vi "Single Tone Audio Measurements.vi"(6 "units settings":T1, 8 "error in":errorcluster, 10 "measurement settings":T4={"Band start"=20.0, "Band stop"=20000.0, "Amplitude"=1.0, "Frequency"=1000.0, "Full scale range"=3.16, "Channel name"="0L"}, 11 "waveform":waveform(dbl)) -> (0 "error out":errorcluster, 1 "spectrum":cluster{"x0":dbl, "dx":dbl, "magnitude":dbl[]}, 2 "time domain":waveform(dbl), 3 "results":T5)   [LabVIEW 2021]
uses:
  controls/single tone audio measurements.ctl
  controls/single tone audio measurement settings.ctl
  <vilib>/addons/_NISVFA/_Shared subVIs/Common/SVL Set dB Reference (variant).vi
  <vilib>/addons/_NISVFA/_Spectrum Processing/SVFA Get Spectrum Subset.vi
  <vilib>/addons/_NISVFA/_Spectrum Processing/SVFA Get Spectrum Subset (Complex) (1 Ch).vi
  <vilib>/addons/_NISVFA/_Shared subVIs/Common/svc_Window Parameters.vi
  <vilib>/addons/_NISVFA/_Shared subVIs/Common/svc_Extract Single Tone Information (complex).vi
  <vilib>/addons/_NISVFA/_Shared subVIs/Common/svc_Check Frequency Range in Spectrum.vi
  <vilib>/addons/_NISVFA/_Spectrum Processing/SVFA Spectrum Peak Search.vi
  <vilib>/addons/_NISVFA/_Spectrum Processing/SVFA Spectrum Peak Search (1 Ch).vi
  <vilib>/addons/_NISVFA/_Shared subVIs/Common/svc_Spectrum Units.vi
  <vilib>/addons/_NISVFA/_Shared subVIs/Common/svc_Log View for Spectrum (1Ch).vi
  <vilib>/addons/_NISVFA/_Spectrum Processing/SVFA Unit Conversion (1 Ch).vi
  <vilib>/addons/_NISVFA/_Shared subVIs/Common/svc_Complex Datatype Defaults.vi
  <vilib>/addons/_NISVFA/_Shared subVIs/Common/svc_Build Unit Label for Frequency Range.vi
  <vilib>/addons/_NISVFA/_Spectrum Processing/SVFA Get Tone Amplitude and Phase (1 Ch).vi
  <vilib>/addons/_NISVFA/_Spectrum Processing/subVIs/svfa_Compute Complex Spectrum for Export.vi
  <vilib>/addons/_NISVFA/_Shared subVIs/Common/svc_Check Frequency Range in Bandwidth.vi
  <vilib>/addons/_NISVFA/_Shared subVIs/Common/svc_Convert Start and Stop to Start Index and Length.vi
  <vilib>/addons/_NISVFA/_Spectrum Processing/subVIs/svfa_Spectrum Peak Search.vi
  <vilib>/addons/_NISVFA/_Shared subVIs/Common/svc_Format Value (DBL).vi
  <vilib>/addons/_NISVFA/_Shared subVIs/Common/svc_Get Weighting Enum and Labels.vi
  <vilib>/addons/_NISVFA/_Shared subVIs/Common/svc_Engineering Units to Unit Label.vi
  <vilib>/addons/_NISVFA/_Shared subVIs/Common/svc_Surround NonAlpha String with Parentheses.vi
  <vilib>/dlg_ctls.llb/Space Constant.vi
  <vilib>/addons/_NISVFA/_Shared subVIs/Common/svc_Unwrap Phase.vi
  <vilib>/addons/_NISVFA/_Shared subVIs/Common/svc_Convert Spectrum Array to dB.vi
  <vilib>/addons/_NISVFA/_Spectrum Processing/subVIs/svfa_Conversion Utility (spectrum info).vi
  <vilib>/addons/_NISVFA/_Spectrum Processing/subVIs/svfa_Window Frequency Response.vi
  <vilib>/addons/_NISVFA/_Spectrum Processing/subVIs/svfa_Window Frequency Response (double array).vi
  <vilib>/Analysis/baseanly.llb/Dot Product.vi
  <vilib>/Analysis/baseanly.llb/Complex Dot Product.vi
  <vilib>/addons/_NISVFA/_Spectrum Processing/subVIs/svfa_Peak Rough Search Indices.vi
  <vilib>/addons/_NISVFA/_Shared subVIs/Common/svc_Unit Label Lexical Class.vi
  <vilib>/addons/_NISVFA/_Spectrum Processing/subVIs/svfa_Peak to RMS to Peak2Peak.vi
  <vilib>/addons/_NISVFA/_Spectrum Processing/subVIs/svfa_Mag to Mag2.vi
  <vilib>/addons/_NISVFA/_Spectrum Processing/subVIs/svfa_Linear to dB.vi
  <vilib>/addons/_NISVFA/_Spectrum Processing/subVIs/svfa_dBrefA to dBrefB.vi
  <vilib>/addons/_NISVFA/_Spectrum Processing/subVIs/svfa_Spectrum to Spectral Density.vi
  <vilib>/addons/_NISVFA/_Spectrum Processing/subVIs/svfa_Rect Window Frequency Response.vi
  <vilib>/addons/_NISVFA/_Spectrum Processing/subVIs/svfa_Cosine Window Coefficients.vi
  <vilib>/addons/_NISVFA/_Shared subVIs/Common/svc_Caller VI Returned in Error Source.vi
  <vilib>/addons/Sound and Vibration/svt_Distortion/subVIs/sv_Check Data Valid (Audio) (1 Ch).vi
  <vilib>/addons/_NISVFA/_Shared subVIs/Common/svc_Convert Frequency to Frequency String.vi
  <vilib>/Analysis/4window.llb/window parameters.vi
  <vilib>/Analysis/4window.llb/Window Properties.vi
  <vilib>/Analysis/4window.llb/Window Properties by Name.vi
  <vilib>/addons/_NISVFA/_Spectrum Processing/subVIs/svfa_Spectrum Peak Tone Search and Estimation (complex).vi
  <vilib>/measure/masignal.llb/Tones and Noise Waveform.vi
  <vilib>/addons/_NISVFA/_Shared subVIs/Common/svc_FFT with Window.vi
  <vilib>/Analysis/1siggen.llb/Square Wave.vi
  <vilib>/addons/_NISVFA/_Spectrum Processing/subVIs/svfa_Three Finger Peak Search.vi
  <vilib>/addons/Sound and Vibration/svt_Distortion/subVIs/sv_Peak View Amplitude (1 Ch).vi
  <vilib>/addons/Sound and Vibration/svt_Single Tone Measurements/SVT Gain (Time) (1 Ch).vi
  <vilib>/addons/Sound and Vibration/svt_Distortion/SVT SNR without Harmonics (Frequency) (1 Ch).vi
  <vilib>/addons/_NISVFA/_Shared subVIs/Common/SVL Set dB Reference (1 Ch).vi
  <vilib>/addons/_NISVFA/_Spectrum Processing/SVFA Unit Conversion (Complex) (1 Ch).vi
  <vilib>/addons/Sound and Vibration/svt_Single Tone Measurements/SVT Spurious Free Dynamic Range (Frequency) (1 Ch).vi
  <vilib>/addons/Sound and Vibration/svt_Single Tone Measurements/SVT Dynamic Range (Frequency) (1 Ch).vi
  <vilib>/addons/Sound and Vibration/svt_Single Tone Measurements/SoundVib_SingleTone.lvlib
  <vilib>/addons/Sound and Vibration/svt_Distortion/SoundVib_Distortion.lvlib
  controls/audio controls.lvlib
  controls/units - ratio.ctl
  controls/units - snr.ctl
  controls/units settings.ctl
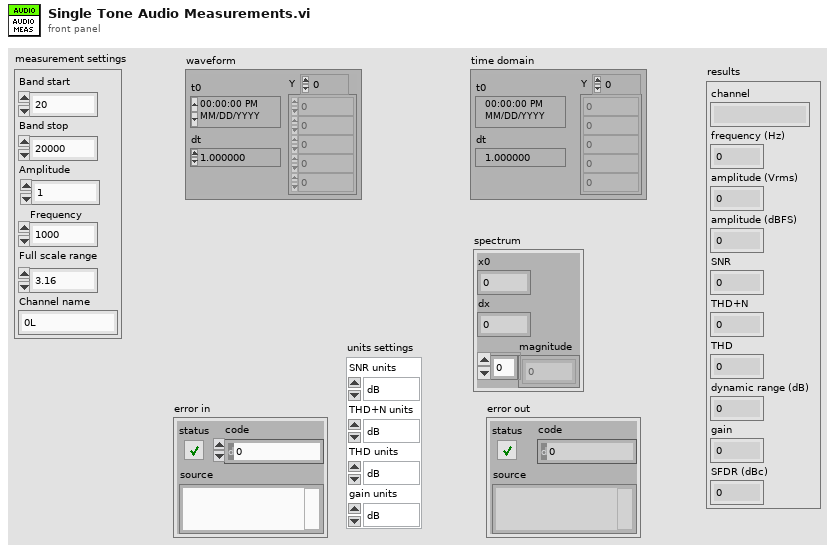
[diagram p1: front panel]
types:
  T1 = typedef "audio controls.lvlib/units settings.ctl" = cluster{"SNR units":T2, "THD+N units":T3, "THD units":T3, "gain units":T3}
  T2 = typedef "audio controls.lvlib/units - snr.ctl" = enum16{"dB", "x/y"}
  T3 = typedef "audio controls.lvlib/units - ratio.ctl" = enum16{"dB", "%", "x/y", "ppm"}
  T4 = typedef "audio controls.lvlib/single tone audio measurement settings.ctl" = cluster{"Band start":dbl, "Band stop":dbl, "Amplitude":dbl, "Frequency":dbl, "Full scale range":dbl, "Channel name":string}
  T5 = typedef "audio controls.lvlib/single tone audio measurements.ctl" = cluster{"channel":string, "frequency (Hz)":dbl, "amplitude (Vrms)":dbl, "amplitude (dBFS)":dbl, "SNR":dbl, "THD+N":dbl, "THD":dbl, "dynamic range (dB)":dbl, "gain":dbl, "SFDR (dBc)":dbl}
  T6 = enum16{"no change", "spectrum", "spectral density"}
  T7 = cluster{"linear/dB":enum16{"no change", "linear", "dB"}, "dB reference (0: no change)":dbl, "power/magnitude":enum16{"no change", "power", "magnitude"}, "view":enum16{"no change", "rms", "peak", "peak-peak"}}
  T8 = cluster{"start frequency":dbl, "stop frequency":dbl}
  T9 = cluster{"gain units":enum16{"dB", "linear ratio"}, "detected fundamental amplitude units":enum16{"EU rms", "EU peak", "EU peak-peak"}}
  T10 = cluster{"SNR units":enum16{"dB", "linear ratio", "%"}, "detected fundamental amplitude units":enum16{"EU rms", "EU peak", "EU peak-peak"}}
  T11 = typedef "svc_Spectrum Info.ctl" = cluster{"channel name":string, "description":string, "x-axis units":T12, "spectral info":cluster{"spectrum type":T13, "linear/dB":enum16{"linear", "dB"}, "window":u16, "window size":i32, "FFT size":i32}, "engineering units":T14, "custom label":string, "dB reference [EU]":dbl, "peak units":enum16{"rms", "peak", "peak-peak"}, "weighting filter":T15, "spectral density?":bool, "unit label":string, "spectrum skewed?":bool, "complimentary spectrum units":T16}
  T12 = typedef "svc_X-Axis Units.ctl" = u16
  T13 = typedef "svc_Spectrum Type.ctl" = enum16{"FFT Spectrum [complex]", "Amplitude [Magnitude]", "Power [Magnitude^2]", "Cross Spectrum [complex]", "Frequency Response [Complex]"}
  T14 = typedef "svc_Engineering Units Text Ring.ctl" = u16
  T15 = typedef "svc_Weighting Filter Text Ring.ctl" = u16
  T16 = typedef "svc_Complimentary Spectrum Units.ctl" = enum16{"none", "radians", "degrees", "cycles", "imaginary"}
  T17 = cluster{"complex spectrum response":cluster{"f0":dbl, "df":dbl, "complex spectrum":cdb[]}, "spectrum info":T11}
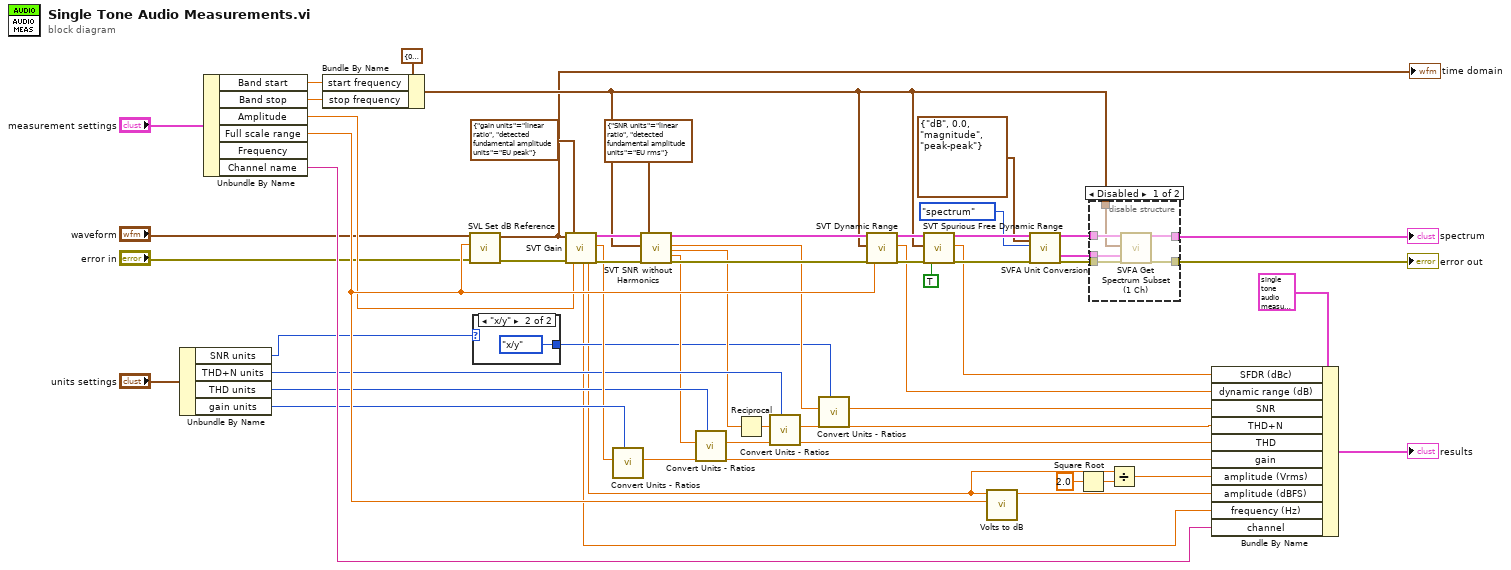
[diagram p0: block diagram]
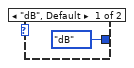
[diagram p2: hidden frame]
diagram:
  n1 = Unbundle By Name("units settings") -> ("SNR units"=w8:T2, "THD+N units"=w17:T3, "THD units"=w11:T3, "gain units"=w20:T3)
  n2 = Unbundle By Name("measurement settings") -> ("Band start"=w54:dbl, "Band stop"=w55:dbl, "Amplitude"=w26:dbl, "Full scale range"=w33:dbl, "Channel name"=w25:string)  [unwired: 1 out]
  n3 = Bundle By Name(cluster=T8 {"start frequency"=0.0, "stop frequency"=0.0} ("frequency range"), "start frequency"=w54, "stop frequency"=w55) -> (w38:T8)
  n4 = call-poly <vilib>:"SVL Set dB Reference.vi"("error in (no error)"="error in", "dB reference [EU]"=w33, "scaled signal in [EU]"="waveform") -> ("error out"=w27:errorcluster, "scaled signal out [EU]"=w23:waveform(dbl))  [unwired: 7 in]
  "time domain" <- w23
  n5 = case shown="\"x/y\"" w8 {
    tunnel: [units_-_ratio."dB" ("gain units") units_-_ratio."x/y" ("gain units")] -> w7
    frame "dB", Default {
    }
    frame "x/y" {
    }
  }
  n6 = call-poly <vilib>:"SVT Gain.vi"("scaled signal [EU]"=w23, "error in (no error)"=w27, "desired units"=T9 {"gain units"=enum."linear ratio", "detected fundamental amplitude units"=enum."EU peak"}, "amplitude [EU peak]"=w26) -> ("detected fundamental\nfrequency [Hz]"=w6:dbl, "detected fundamental\namplitude"=w1:dbl, "complex spectrum"=w44:T17, "gain"=w19:dbl, "error out"=w45:errorcluster)  [unwired: 10 in, 1 out]
  n7 = call "Convert Units - Ratios.vi"("gain units"=w20, "linear ratio"=w19) -> ("converted ratio"=w18:dbl)  [unwired: 9 in]
  n8 = call-poly <vilib>:"SVT SNR without Harmonics.vi"("complex spectrum"=w44, "frequency range"=w38, "error in (no error)"=w45, "desired units"=T10 {"SNR units"=enum."linear ratio", "detected fundamental amplitude units"=enum."EU rms"}) -> ("complex spectrum"=w47:T17, "SNR (without harmonics)"=w16:dbl, "SINAD"=w13:dbl, "THD"=w10:dbl, "error out"=w46:errorcluster)  [unwired: 8 in, 3 out]
  n9 = call "Convert Units - Ratios.vi"("gain units"=w11, "linear ratio"=w10) -> ("converted ratio"=w9:dbl)  [unwired: 9 in]
  n10 = Reciprocal(x=w13) -> (1/x=w14:dbl)
  n11 = call "Convert Units - Ratios.vi"("gain units"=w17, "linear ratio"=w14) -> ("converted ratio"=w12:dbl)  [unwired: 9 in]
  n12 = call "Convert Units - Ratios.vi"("gain units"=w7, "linear ratio"=w16) -> ("converted ratio"=w15:dbl)  [unwired: 9 in]
  n13 = call-poly <vilib>:"SVT Dynamic Range.vi"("complex spectrum"=w47, "frequency range"=w38, "error in (no error)"=w46, "full scale amplitude [EU peak]"=w33) -> ("dup complex spectrum"=w50:T17, "dynamic range"=w31:dbl, "error out"=w51:errorcluster)  [unwired: 10 in, 3 out]
  n14 = call-poly <vilib>:"SVT Spurious Free Dynamic Range.vi"("complex spectrum"=w50, "frequency range"=w38, "error in (no error)"=w51, "exclude harmonics"=TRUE) -> ("complex spectrum"=w42:T17, "spurious free dynamic range"=w32:dbl, "error out"=w43:errorcluster)  [unwired: 8 in, 5 out]
  n15 = call "Volts to dB.vi"("Full scale range"=w33, "Voltage(V)"=w1) -> ("Voltage(dB)"=w5:dbl)  [unwired: 9 in]
  n16 = call-poly <vilib>:"SVFA Unit Conversion.vi"("complex spectrum"=w42, "desired scaling"=T7 {"linear/dB"=enum."dB", "dB reference (0: no change)"=0.0, "power/magnitude"=enum."magnitude", "view"=enum."peak-peak"}, "spectral density desired"=T6."spectrum", "error in (no error)"=w43) -> ("converted spectrum"=w39:cluster{"x0":dbl, "dx":dbl, "magnitude":dbl[]}, "spectrum info out"=w36:T11, "error out"=w35:errorcluster)  [unwired: 10 in, 3 out]
  n17 = Square Root(x=2.0 ("y")) -> (sqrt(x)=w4:dbl)
  n18 = disable-structure shown="Disabled" {
    disable-tunnel: w39 -> [w63 w64]
    disable-tunnel: w38 -> [w62 _]
    disable-tunnel: [w61 w65] -> w37
    disable-tunnel: w36 -> [w60 _]
    disable-tunnel: w35 -> [w59 w65]
    disable-tunnel: [w58 w64] -> w28
    frame Disabled {
      n19 = call <vilib>:"SVFA Get Spectrum Subset (1 Ch).vi"("spectrum"=w63, "range"=w62, "spectrum info"=w60, "error in (no error)"=w59) -> ("spectrum subset"=w58:cluster{"x0":dbl, "dx":dbl, "magnitude":dbl[]}, "error out"=w61:errorcluster)  [unwired: 10 in, 4 out]
    }
    frame Enabled {
    }
  }
  "error out" <- w37
  "spectrum" <- w28
  n20 = Divide(x=w1, y=w4) -> (x/y=w2:dbl)
  n21 = Bundle By Name(cluster=T5 {"channel"="", "frequency (Hz)"=0.0, "amplitude (Vrms)"=0.0, "amplitude (dBFS)"=0.0, "SNR"=0.0, "THD+N"=0.0, "THD"=0.0, "dynamic range (dB)"=0.0, "gain"=0.0, "SFDR (dBc)"=0.0} ("results"), "SFDR (dBc)"=w32, "dynamic range (dB)"=w31, "SNR"=w15, "THD+N"=w12, "THD"=w9, "gain"=w18, "amplitude (Vrms)"=w2, "amplitude (dBFS)"=w5, "frequency (Hz)"=w6, "channel"=w25) -> (→"results":T5)
